vi "FRCts20_Backend_InitializeDates.vi"(8 "error in (no error)":errorcluster, 11 "XML Parent":path) -> (0 "error out":errorcluster)   [LabVIEW 2013, in "FRCts20_Backend_Engine_Deprecated.lvlib"]
doc: "Reads competition dates from INI and stores them in the data line."
uses:
  FRCts20_Backend_Engine_Deprecated.lvlib
  FRCts20_Backend_FGVDatesCommands.ctl
  <vilib>/Utility/config.llb/Read Key (String).vi
  <vilib>/Utility/config.llb/Write Key (String).vi
  <vilib>/Utility/config.llb/NI_LVConfig.lvlib
  FRCts20_Backend_Controls.lvlib
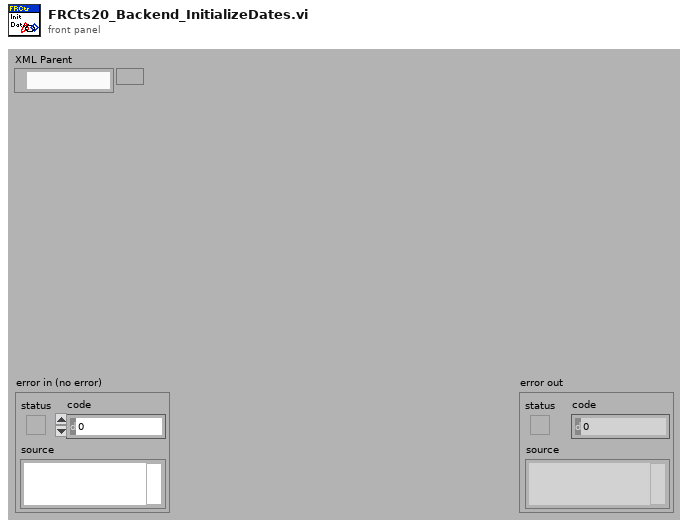
[diagram p1: front panel]
types:
  T1 = typedef "FRCts20_Backend_Controls.lvlib/FRCts20_Backend_FGVDatesCommands.ctl" = enum16{"Set Dates", "Get Day", "Get First Day"}
  T2 = typedef "NI_LVConfig.lvlib/Config Data RefNum.ctl" = refnum<k1>
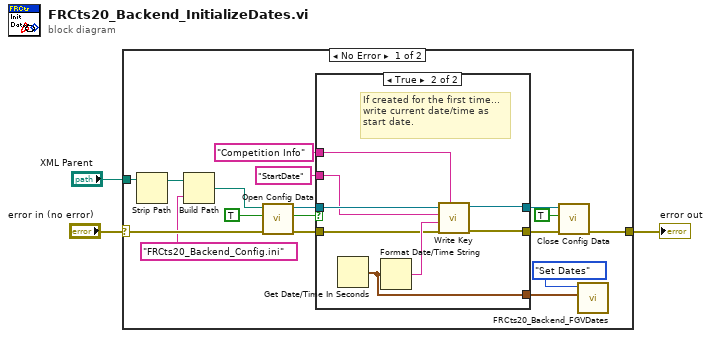
[diagram p0: block diagram]
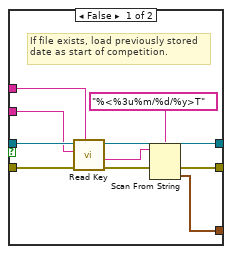
[diagram p2: hidden frame]
diagram:
  n1 = case shown="No Error" "error in (no error)" {
    selector: "error in (no error)" -> [w18 w39]
    tunnel: [w7 w39] -> w2
    tunnel: "XML Parent" -> [w20 _]
    frame No Error {
      n2 = Strip Path(path=w20) -> (stripped path=w6:path)  [unwired: 1 out]
      n3 = Build Path(base path=w6, name or relative path="FRCts20_Backend_Config.ini") -> (appended path=w4:path)
      n4 = call <vilib>:"Open Config Data.vi"("error in (no error)"=w18, "create file if necessary (T)"=TRUE, "configuration file path"=w4) -> ("error out"=w16:errorcluster, "file created?"=w17:bool, "refnum"=w15:T2)  [unwired: 6 in]
      n5 = case shown="True" w17 {
        tunnel: w16 -> [w30 w36]
        tunnel: w15 -> [w29 w38]
        tunnel: "StartDate" ("section") -> [w27 w35]
        tunnel: "Competition Info" ("section") -> [w28 w34]
        tunnel: [w23 w33] -> w12
        tunnel: [w24 w31] -> w9
        tunnel: [w22 w32] -> w10
        frame False {
          # "If file exists, load previously stored\ndate as start of competition."
          n6 = call-poly <vilib>:"Read Key.vi"("section"=w28, "error in (no error)"=w30, "key"=w27, "refnum"=w29) -> ("error out"=w26:errorcluster, "value"=w25:string, "refnum out"=w24:T2)  [unwired: 4 in, 1 out]
          n7 = Scan From String(format string="%<%3u%m/%d/%y>T", input string=w25, error in=w26) -> (error out=w22:errorcluster, output 1=w23:timestamp)  [unwired: 2 in, 2 out]
        }
        frame True {
          # "If created for the first time...\nwrite current date/time as \nstart date."
          n8 = Get Date/Time In Seconds() -> (seconds since 1Jan1904=w33:timestamp)
          n9 = Format Date/Time String(seconds (now)=w33) -> (date/time string=w37:string)  [unwired: 2 in]
          n10 = call-poly <vilib>:"Write Key.vi"("section"=w34, "error in (no error)"=w36, "value"=w37, "key"=w35, "refnum"=w38) -> ("error out"=w32:errorcluster, "refnum out"=w31:T2)  [unwired: 4 in, 1 out]
        }
      }
      n11 = call <vilib>:"Close Config Data.vi"("error in (no error)"=w10, "write file if changed (T)"=TRUE, "refnum"=w9) -> ("error out"=w7:errorcluster)  [unwired: 7 in, 1 out]
      n12 = call "FRCts20_Backend_FGVDates.vi"("Date"=w12, "Command"=FRCts20_Backend_FGVDatesCommands."Set Dates") -> ()  [unwired: 7 in, 3 out]
    }
    frame Error {
    }
  }
  "error out" <- w2
